vi "PID Engine Settle Timer BAP5.vi"(8 "Control Parameters":T1 {"Settle time" format="%.2f"; "Derivative time" format="%.2f"; "Integral time" format="%.2f"; "Settle bandwidth" format="%.2f"; "Control bandwidth" format="%.2f"; "Setpoint" format="%.2f"}, 9 "RESET":bool, 10 "elapsed time":dbl, 11 "Temp In (deg C)":dbl) -> (1 "settled":bool, 2 "time in settle band":dbl)   [LabVIEW 2014]
doc: "PID Engine Settle Timer BAP5\n\nReturns the Time in the Settled Band (s) and if the Temperature is settled based of the Settle Time (s), Setpoint(°C), Settle Bandwidth (°C), Current Temperature (°C), Elapsed Time (s), and RESET. RESET initializes previous time in settle band to 0.\n\nTime in Settle Band = Previous Time in Settle Band + Elapsed Time, if it is within the range of the settle band limits. \n = 0, otherwise\n\nTemperature is settled if Time in Settle Band is greater than or equal to Settle Time.\n\nBeverly Abadines\nPHY 350"
uses:
  typedefs/control parameters.ctl
panel:
  # "PID Engine Settle Timer"
  # "Beverly Abadines\nPhys 350\nP5"
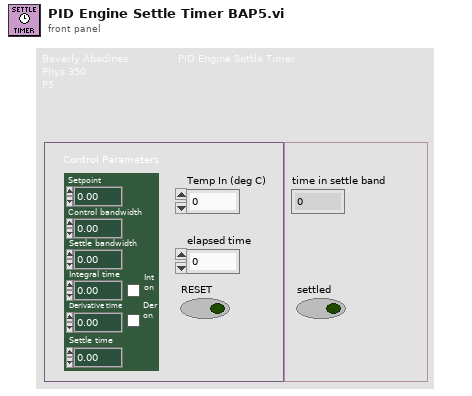
[diagram p1: front panel]
types:
  T1 = typedef "control parameters.ctl" = cluster{"Setpoint":dbl, "Control bandwidth":dbl, "Settle bandwidth":dbl, "Integral time":dbl, "Int\non":bool, "Derivative time":dbl, "Der\non":bool, "Settle time":dbl}
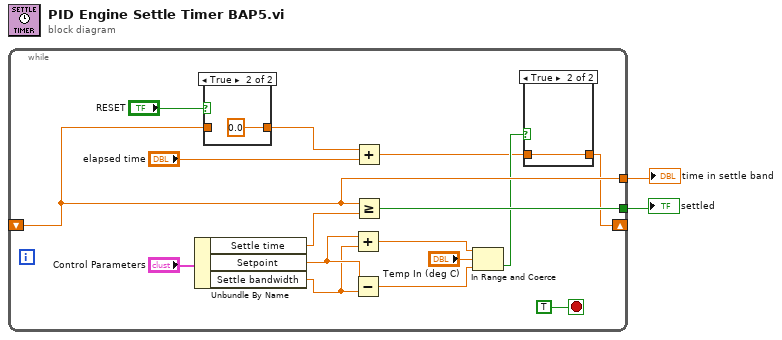
[diagram p0: block diagram]
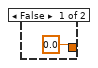
[diagram p2: hidden frame]
diagram:
  n1 = while {
    shift-right: [w3] -> _
    shift-left: _ -> [w6]
    tunnel: [w7] -> w2
    tunnel: [w6] -> w1
    stop <- TRUE stop-if-true
    n2 = Unbundle By Name("Control Parameters") -> ("Settle time"=w8:dbl, "Setpoint"=w17:dbl, "Settle bandwidth"=w16:dbl)
    n3 = case shown="True" "RESET" {
      tunnel: w6 -> [w21 _]
      tunnel: [w21 0.0] -> w10
      frame False {
      }
      frame True {
      }
    }
    n4 = Add(x=w17, y=w16) -> (x+y=w12:dbl)
    n5 = Subtract(x=w17, y=w16) -> (x-y=w11:dbl)
    n6 = Add(x=w10, y="elapsed time") -> (x+y=w4:dbl)
    n7 = Greater Or Equal?(x=w6, y=w8) -> (x >= y?=w7:bool)
    n8 = In Range and Coerce(upper limit=w12, x="Temp In (deg C)", lower limit=w11) -> (In Range?=w5:bool)  [unwired: 1 out]
    n9 = case shown="True" w5 {
      tunnel: w4 -> [_ w20]
      tunnel: [0.0 w20] -> w3
      frame False {
      }
      frame True {
      }
    }
  }
  "settled" <- w2
  "time in settle band" <- w1
